vi "Fetch Waveforms.vi"(8 "error in":errorcluster, 11 "HDO4000A Base CFG in":refnum<class "HDO4000A Base CFG.lvclass">) -> (0 "error out":errorcluster, 2 "Last Waveforms":map{u8, waveform(dbl)}(c390), 3 "HDO4000A Base CFG out":refnum<class "HDO4000A Base CFG.lvclass">)   [LabVIEW 2023]
uses:
  HDO4000A Base CFG.lvclass
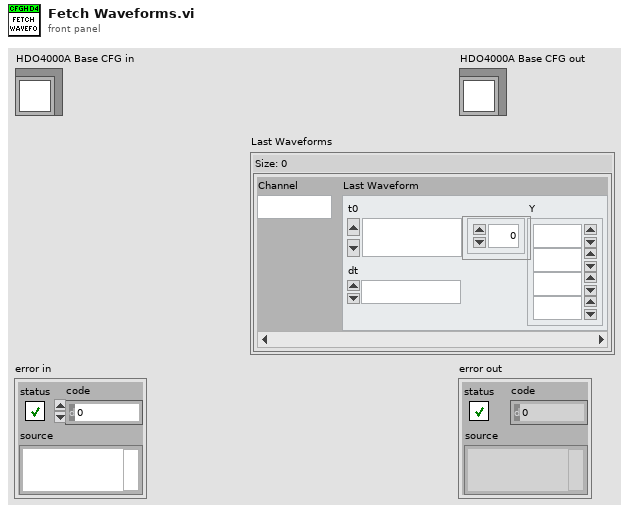
[diagram p1: front panel]
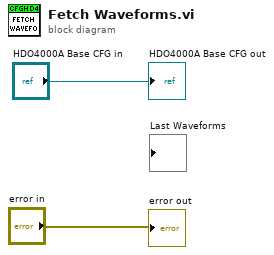
[diagram p0: block diagram]
diagram:
  "error out" <- "error in"
  "HDO4000A Base CFG out" <- "HDO4000A Base CFG in"
